vi "TestResizeGreyscaleImage.vi"(8 "error in (no error)":errorcluster, 11 "Test Case In":refnum<class "Image.lvclass">) -> (0 "error out":errorcluster, 3 "Test Case Out":refnum<class "Image.lvclass">)   [LabVIEW 2020, in "g_ar_toolkit.test.lvlib" / "Image.lvclass"]
uses:
  Image.lvclass
  C:/Program Files (x86)/National Instruments/LabVIEW 2020/vi.lib/Astemes/LUnit/Test Case.lvclass
  g_ar_toolkit/Image Size Cluster.ctl
  g_ar_toolkit/OpenCV Interpolation Enum.ctl
  <vilib>/Astemes/LUnit/Test Case.lvclass/Test Case.ctl
  g_ar_toolkit/Create_Empty_Image_Greyscale.vi
  g_ar_toolkit/Resize_RetainData_Greyscale.vi
  4993e8ee-a06a-463a-9684-69129f64d5ce.vi
  g_ar_toolkit/ResizeCore_Greyscale.vi
  <vilib>/Astemes/LUnit/Append Pass Result.vi
  <vilib>/Astemes/LUnit/Append Fail Result.vi
  <vilib>/Astemes/LUnit/Describe Comparison.vi
  <vilib>/Astemes/LUnit/Compare Variants.vi
  <vilib>/Astemes/LUnit/Variant to string.vi
  <vilib>/Utility/error.llb/Error Cluster From Error Code.vi
  <vilib>/Utility/Data Type/Get Type Information.vi
  <vilib>/Utility/LVClass/Get LV Class Name.vi
  g_ar_toolkit.lvlib
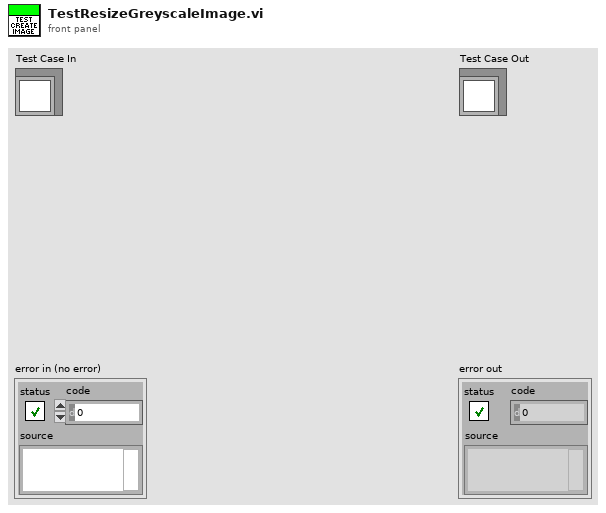
[diagram p1: front panel]
types:
  T1 = typedef "g_ar_toolkit.lvlib/OpenCV Interpolation Enum.ctl" = enum16{"NEAREST", "LINEAR", "CUBIC", "AREA", "LANCZOS", "LINEAR_EXACT", "NEAREST_EXACT", "MAX"}
  T2 = typedef "g_ar_toolkit.lvlib/Image Size Cluster.ctl" = cluster{"Width":u16, "Height":u16}
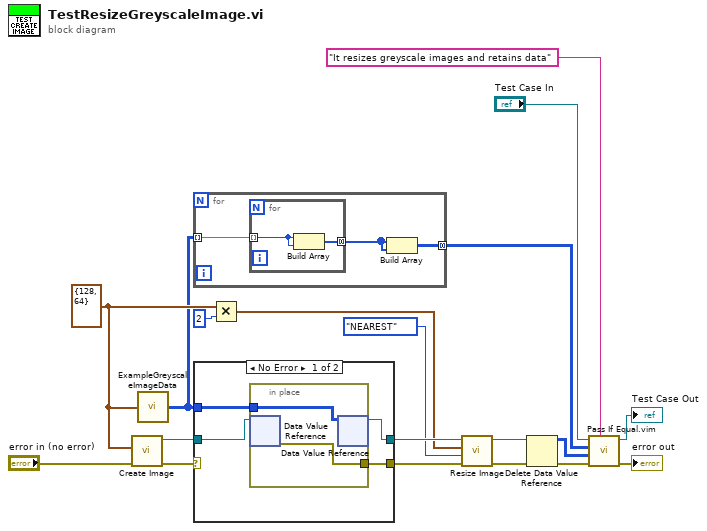
[diagram p0: block diagram]
diagram:
  w6 = T2 {"Width"=128, "Height"=64} ("Preallocated Image Size (Default - 0,0)")
  n1 = call-poly "Create Image.vi"("error in (no error)"="error in (no error)", "Preallocated Image Size (Default 0,0)"=w6) -> ("error out"=w13:errorcluster, "New Greyscale Image"=w12:refnum<data-value>)  [unwired: 8 in]
  n2 = call "ExampleGreyscaleImageData.vi"("Image Size"=w6) -> ("GreyscaleImage"=w2:u8[][])
  n3 = for {
    tunnel: w2 -> [w22] mode=indexing
    tunnel: [w20] -> w1 mode=concatenating
    n4 = for {
      tunnel: w22 -> [w24] mode=indexing
      tunnel: [w23] -> w21 mode=concatenating
      n5 = Build Array(w24, w24) -> (w23:u8[])
    }
    n6 = Build Array(w21, w21) -> (w20:u8[][])
  }
  n7 = case shown="No Error" w13 {
    selector: w13 -> [_ w31]
    tunnel: w12 -> [w28 w32]
    tunnel: w2 -> [w27 _]
    tunnel: [w26 w32] -> w10
    tunnel: [w25 w31] -> w9
    frame No Error {
      n8 = in-place {
        in-place-border: w27 -> [w30]
        in-place-border: [w29] -> w25
        n9 = in-place-dvr #1(w28) -> (w29:errorcluster)  [unwired: 1 out]
        n10 = in-place-dvr #1(w30) -> (w26:refnum<data-value>)  [unwired: 1 out]
      }
    }
    frame Error {
    }
  }
  n11 = Multiply(x=w6, y=u16 2) -> (x*y=w4:T2)
  n12 = call-poly "Resize Image.vi"("error in (no error)"=w9, "OpenCV Interpolation Flag"=OpenCV_Interpolation_Enum."NEAREST", "New Image Size"=w4, "Greyscale Image"=w10) -> ("error out"=w7:errorcluster, "Greyscale Image (duplicate)"=w8:refnum<data-value>)  [unwired: 6 in]
  n13 = Delete Data Value Reference(data value reference=w8, error in=w7) -> (data value=w11:u8[][], error out=w15:errorcluster)
  n14 = call "Pass If Equal.vim"("Description"="It resizes greyscale images and retains data", "error in (no error)"=w15, "Actual"=w11, "Expected"=w1, "LUnit Test Case In"="Test Case In") -> ("error out"=→"error out":errorcluster, "LUnit Test Case Out"=→"Test Case Out":refnum<class "Image.lvclass">)  [unwired: 5 in]
